vi "Two Buttons Dialog Window.vi"(1 "Cancel Button Text":string="Cancel", 2 "OK Button Text":string="OK", 3 "Message":string) -> (0 "OK?":bool)   [LabVIEW 2019]
panel:
  in  "Checkbox":bool
  in  "Cancel":bool
  in  "OK":bool
  out "Displayed Message":string
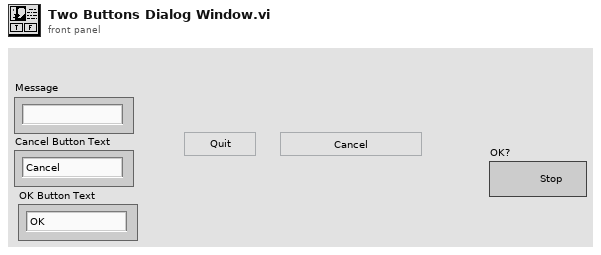
[diagram p1: front panel]
types:
  T1 = cluster{"Displayed Message":refnum<vi>, "Checkbox":refnum<vi>, "Cancel":refnum<vi>, "OK":refnum<vi>}
  T2 = enum32{"Invalid", "Standard", "Closed", "Hidden", "Minimized", "Maximized"}
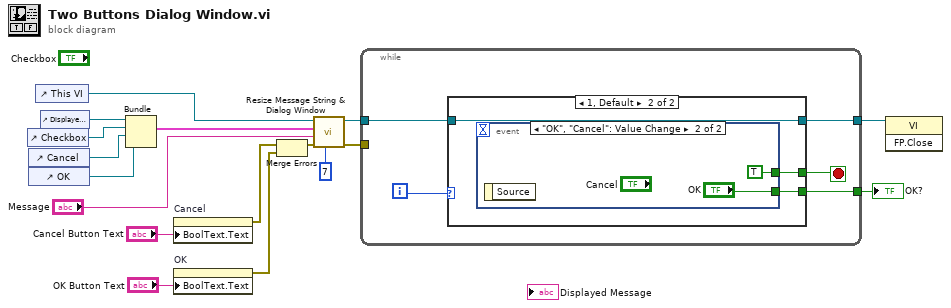
[diagram p0: block diagram]
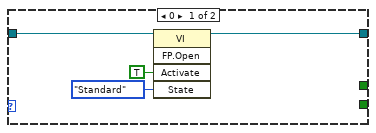
[diagram p2: hidden frame]
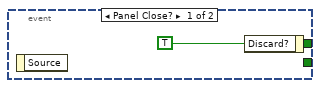
[diagram p3: hidden frame]
diagram:
  n1 = control-ref of="Checkbox"() -> (w5:refnum<vi>)
  n2 = control-ref of="Cancel"() -> (w6:refnum<vi>)
  n3 = control-ref of="OK"() -> (w12:refnum<vi>)
  n4 = control-ref of="This VI"() -> (w11:refnum<vi>)
  n5 = control-ref of="Displayed Message"() -> (w13:refnum<vi>)
  n6 = Bundle("Displayed Message"=w13, "Checkbox"=w5, "Cancel"=w6, "OK"=w12) -> (w10:T1)  [unwired: 1 in]
  n7 = property on="Cancel" class="Bool"("BoolText.Text"="Cancel Button Text") -> (error out=w4:errorcluster)  [unwired: 2 in, 1 out]
  n8 = property on="OK" class="Bool"("BoolText.Text"="OK Button Text") -> (error out=w2:errorcluster)  [unwired: 2 in, 1 out]
  n9 = Merge Errors(w4, w2) -> (w3:errorcluster)
  n10 = call "Resize Message String & Dialog Window.vi"("Max Number of Lines"=7, "Error In"=w3, "Message"="Message", "Controls & Indicators"=w10, "VI Refnum"=w11) -> ("Error Out"=w1:errorcluster, "VI Refnum out"=w7:refnum<vi>)  [unwired: 5 in]
  n11 = while {
    tunnel: w7 -> [w19]
    tunnel: [w18] -> w17
    tunnel: [w21] -> w14
    tunnel: w1 -> [_]
    i -> [w20]
    stop <- w22 stop-if-true
    n12 = case shown="1, Default" w20 {
      tunnel: [_ w29] -> w22
      tunnel: [_ w28] -> w21
      tunnel: w19 -> [w26 w27]
      tunnel: [w25 w27] -> w18
      frame 0 {
        n13 = invoke class="VI" method="FP.Open"(reference=w26, "Activate"=TRUE ("Activate?"), "State"=T2."Standard") -> (reference out=w25:refnum<vi>)  [unwired: 2 in, 4 out]
      }
      frame 1, Default {
        n14 = event shown="[1] \"OK\", \"Cancel\": Value Change" {
          selector: _ -> [_ _]
          dyn-events: _ -> [_ _]
          timeout: _ -> [_ _]
          tunnel: [w30 TRUE ("Discard?")] -> w29
          tunnel: [_ "OK"] -> w28
          event Panel Close? {
            w30 = TRUE ("Discard?")
            n15 = event-data() -> ()  [unwired: 1 in, 1 out]
            n16 = event-data("Discard?"=w30) -> ()  [unwired: 1 in, 1 out]
          }
          event "OK", "Cancel": Value Change {
            n17 = event-data() -> ()  [unwired: 1 in, 1 out]
          }
        }
      }
    }
  }
  "OK?" <- w14
  n18 = invoke class="VI" method="FP.Close"(reference=w17) -> ()  [unwired: 2 in, 3 out]
